vi "mainGUI_looped.vi"() -> ()   [LabVIEW 2025]
uses:
  <vilib>/Utility/error.llb/DialogType.ctl
  <vilib>/DAQmx/write.llb/DAQmx Write (Analog 1D Wfm NChan NSamp).vi
  <vilib>/DAQmx/read.llb/DAQmx Read (Analog Wfm 1Chan NSamp).vi
  <vilib>/DAQmx/read.llb/DAQmx Read (Counter U32 1Chan 1Samp).vi
  <vilib>/DAQmx/miscellaneous.llb/DAQmx Fill In Error Info.vi
  <vilib>/DAQmx/create/channels.llb/DAQmx Create Channel (CI-Count Edges).vi
  <vilib>/DAQmx/configure/trigger.llb/DAQmx Start Trigger (Digital Edge).vi
  <resource>/objmgr/daqmx.rc
  <vilib>/Analysis/NI_AALPro.lvlib
panel:
  in  "Run Live":bool caption="Run live"
  in  "Begin Experiment":bool
  in  "Connect Kinetix":bool
  in  "Run time":i32 caption="s" min=0
  in  "SLM default":bool
  in  "Load SLM image":bool
  in  "Create SLM image":bool
  in  "Save directory":path=path "D:/KinetixTest/SS_test"
  in  "# Trials":u32=1 caption="trials" min=1 step=1
  in  "Trial Time":dbl=0.1 caption="s" min=0.1 max=60.0 format="%#_2g"
  in  "Galvo frequency":u16(ring)=100 caption="Hz" items=["20"=20, "100"=100, "800"=800]
  in  "Galvo voltage":dbl=1.0 caption="V" min=0.1 max=1.8 format="%#_2g"
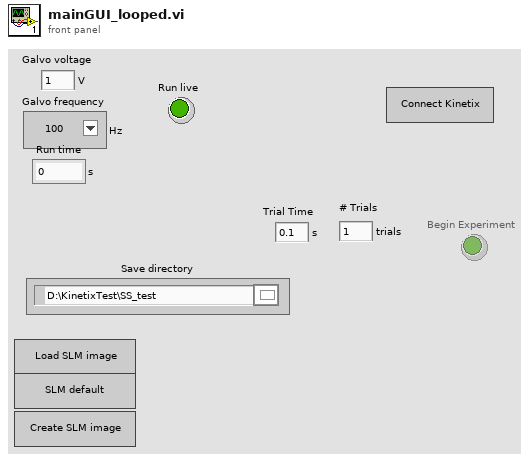
[diagram p1: front panel]
types:
  T1 = enum16{"open", "open or create", "create or replace", "create", "open (read-only)"}
  T2 = typedef "DialogType.ctl" = u16
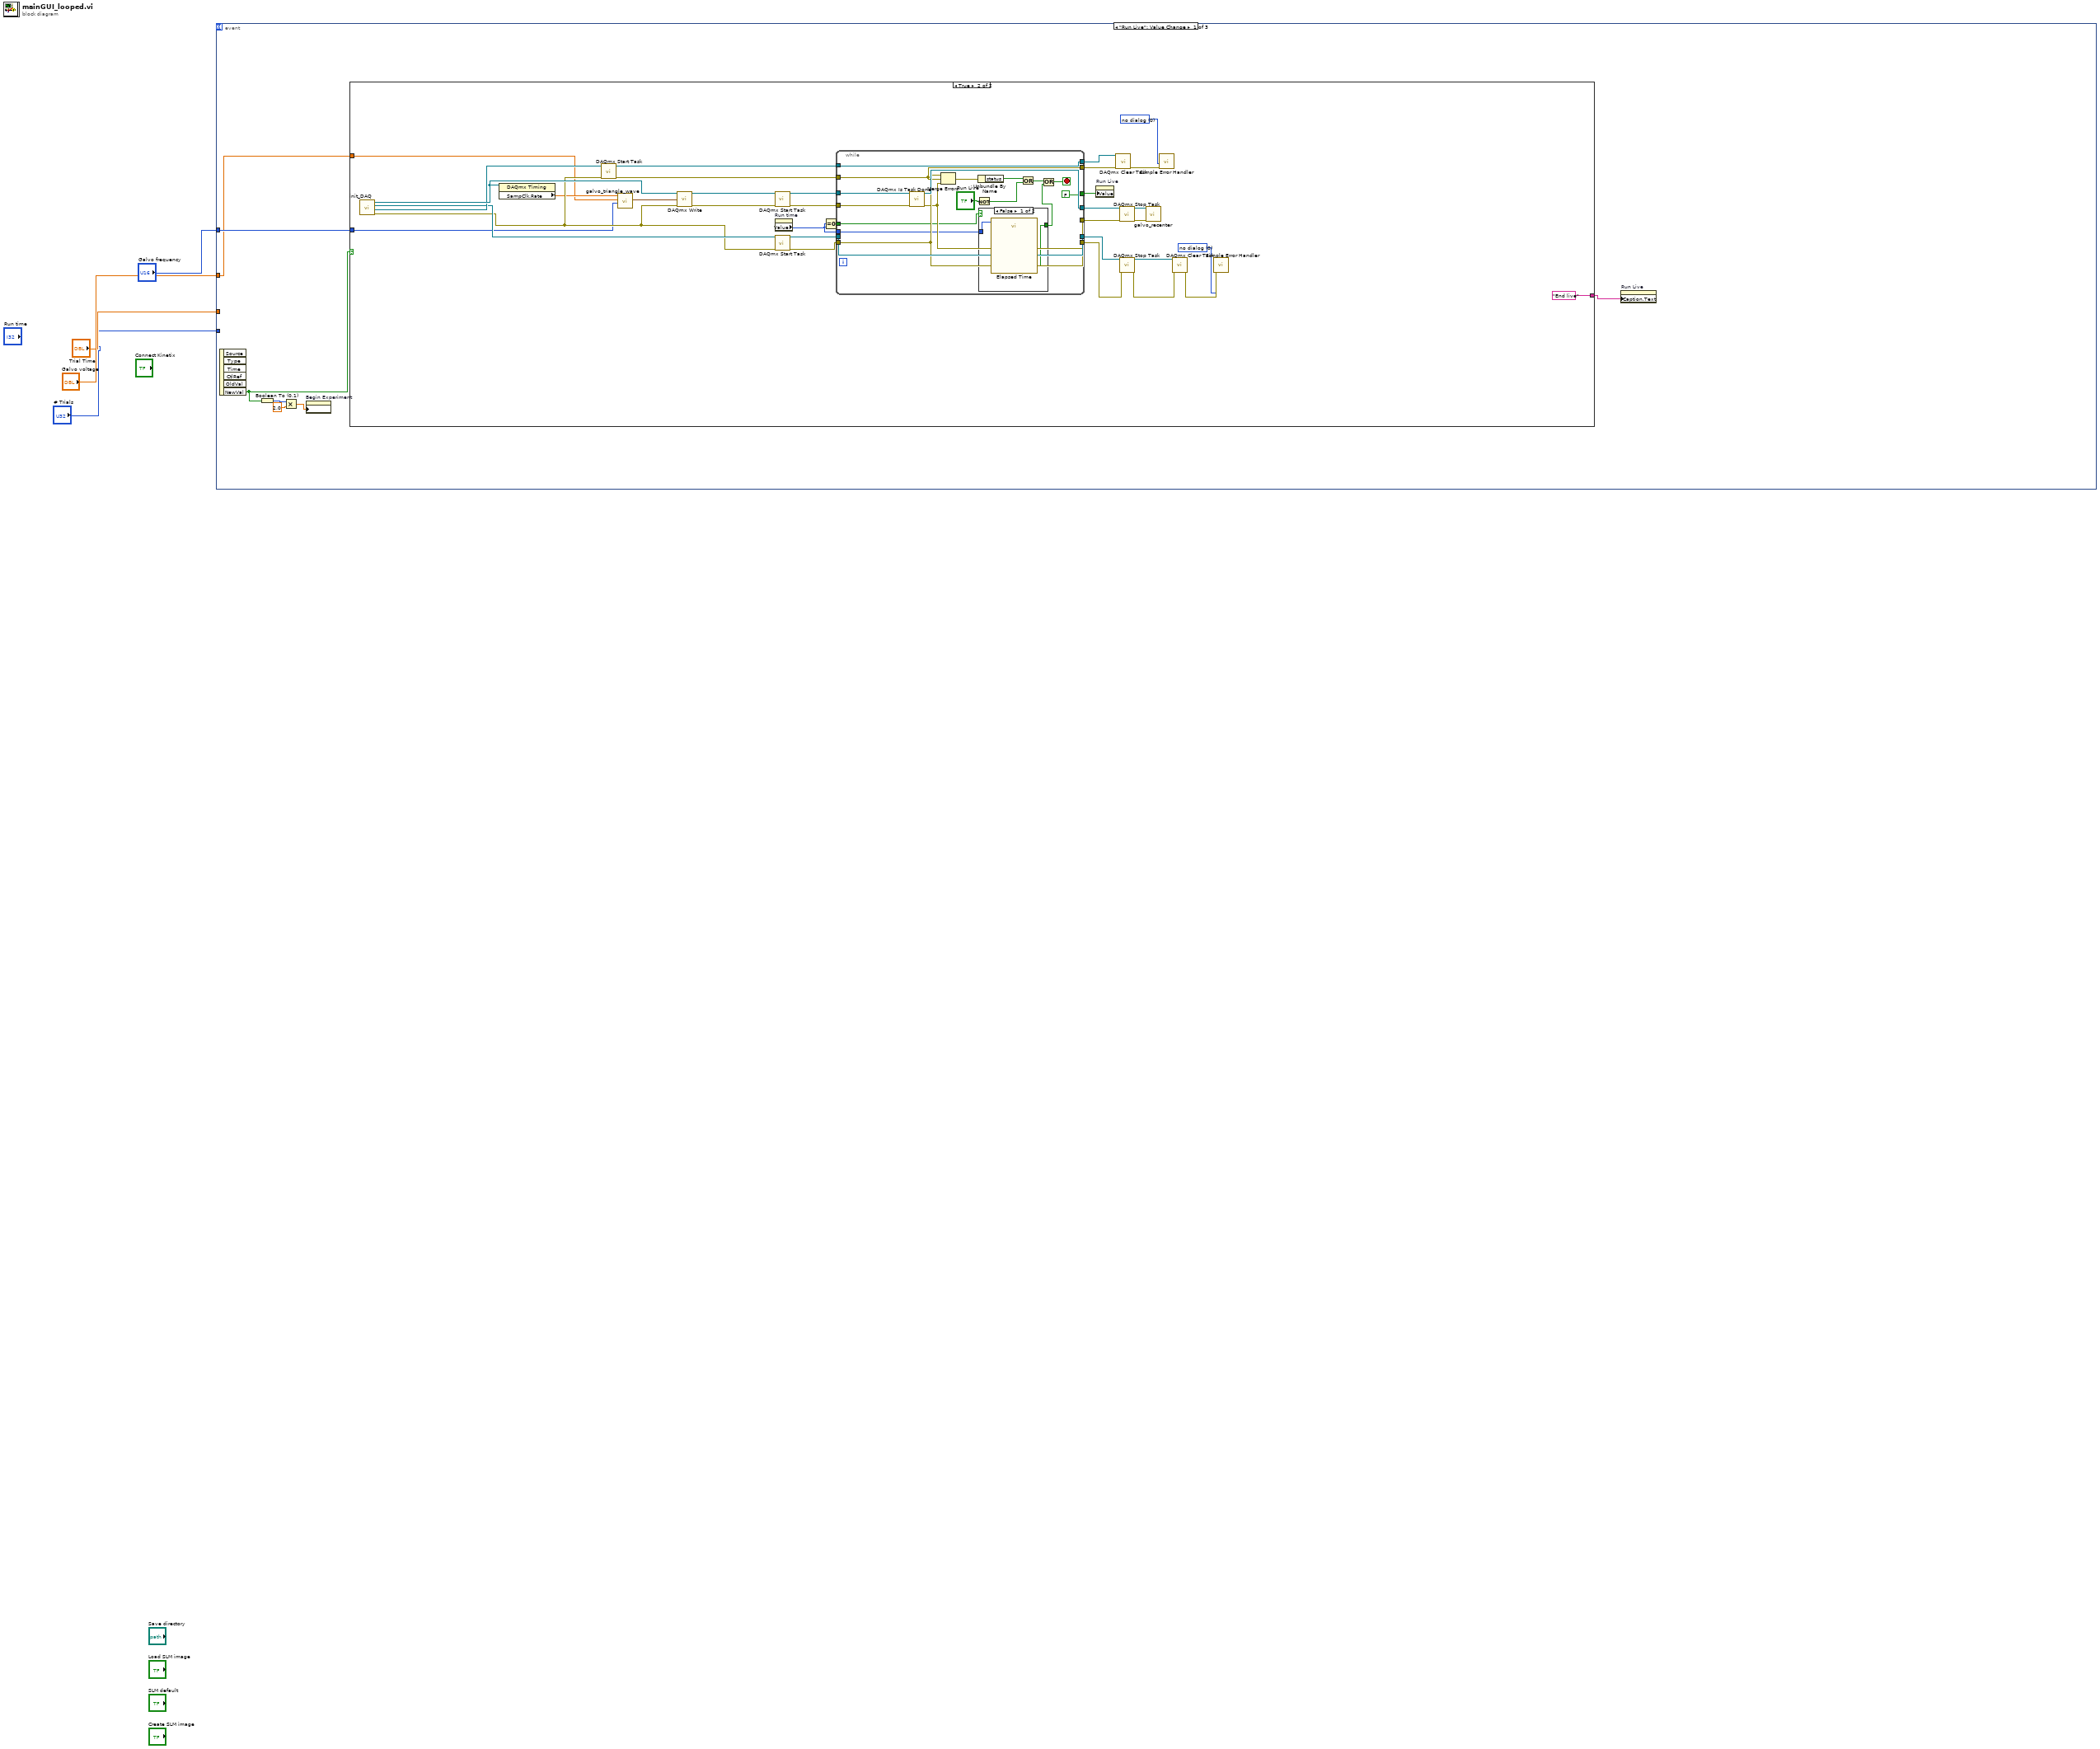
[diagram p0: block diagram]
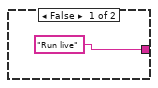
[diagram p2: hidden frame]
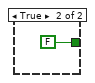
[diagram p3: hidden frame]
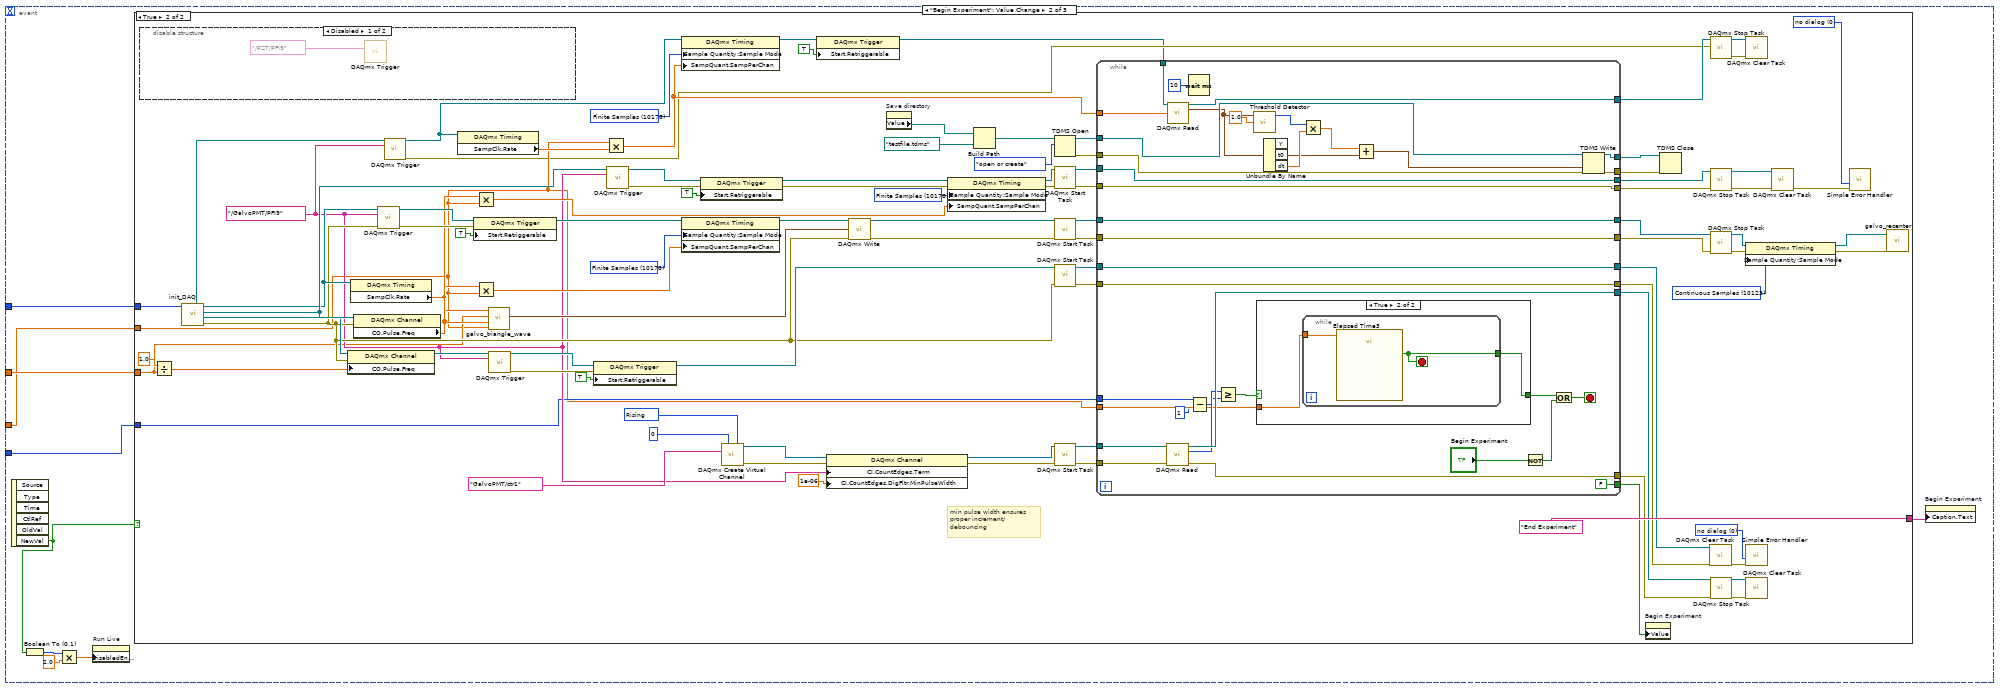
[diagram p4: hidden frame]
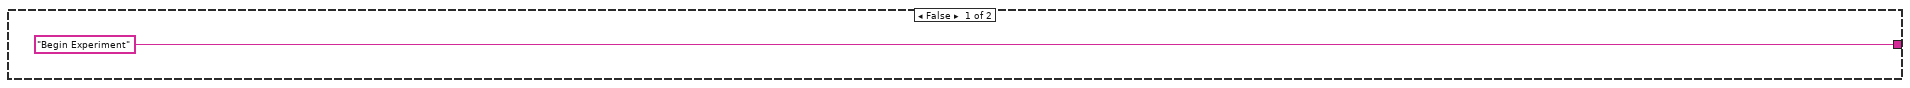
[diagram p5: hidden frame]
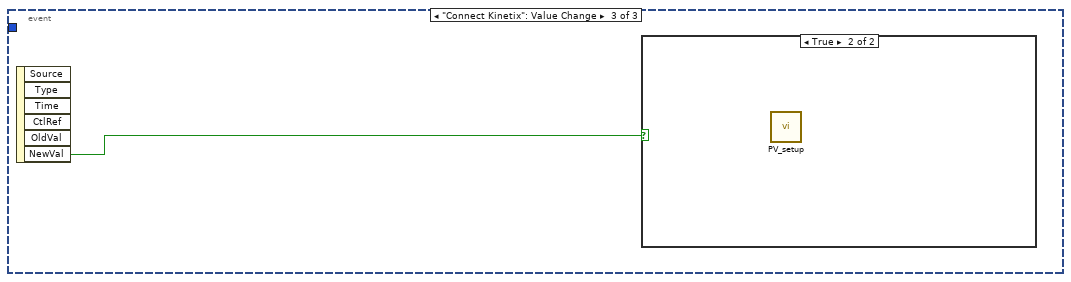
[diagram p8: hidden frame]
diagram:
  n1 = event shown="[0] \"Run Live\": Value Change" {
    selector: _ -> [_ _ _]
    dyn-events: _ -> [_ _ _]
    timeout: _ -> [_ _ _]
    tunnel: "Galvo frequency" -> [w7 w73 _]
    tunnel: "Galvo voltage" -> [w6 w72 _]
    tunnel: "Trial Time" -> [_ w71 _]
    tunnel: "# Trials" -> [_ w70 _]
    event "Run Live": Value Change {
      n2 = event-data() -> ("NewVal"=w5:bool)  [unwired: 1 in, 5 out]
      n3 = Boolean To (0,1)(Boolean=w5) -> (0, 1=w10:i16)
      n4 = Multiply(x=w10, y=2.0) -> (x*y=w9:dbl)
      n5 = property on="Begin Experiment" class="Bool (strict)"("DisabledEnum"=w9) -> ()  [unwired: 2 in, 2 out]
      n6 = case shown="True" w5 {
        tunnel: ["Run live" "End live"] -> w8
        tunnel: w7 -> [_ w14]
        tunnel: w6 -> [_ w13]
        frame False {
        }
        frame True {
          w33 = T2 0 items=["no dialog", "OK message", "continue or stop message", "OK message + warnings", "continue/stop + warnings"] ("type of dialog (OK msg:1)")
          w35 = T2 0 items=["no dialog", "OK message", "continue or stop message", "OK message + warnings", "continue/stop + warnings"] ("type of dialog (OK msg:1)")
          n7 = call "init_DAQ.vi"() -> ("error out"=w22:errorcluster, "shutter trigger task"=w28:refnum<k21>, "Kinetix trigger task"=w23:refnum<k21>, "galvo driving task"=w39:refnum<k21>)  [unwired: 7 in, 1 out]
          n8 = property class="DAQmx Timing"(reference=w39) -> ("SampClk.Rate"=w20:dbl)  [unwired: 1 in, 2 out]
          n9 = call <vilib>:"DAQmx Start Task.vi"("task/channels in"=w28, "error in"=w22) -> ("task out"=w32:refnum<k21>, "error out"=w30:errorcluster)  [unwired: 12 in]
          n10 = call "galvo_triangle_wave.vi"("final frequency"=w14, "amplitude"=w13, "sample rate"=w20) -> ("waveform array out"=w21:waveform(dbl)[])  [unwired: 8 in]
          n11 = call-poly <vilib>:"DAQmx Write.vi"("task/channels in"=w39, "data"=w21, "error in"=w22) -> ("task out"=w45:refnum<k21>, "error out"=w44:errorcluster)  [unwired: 10 in, 1 out]
          n12 = call <vilib>:"DAQmx Start Task.vi"("task/channels in"=w45, "error in"=w44) -> ("task out"=w40:refnum<k21>, "error out"=w41:errorcluster)  [unwired: 12 in]
          n13 = property on="Run time" class="DigNum (strict)"() -> ("Value"=w16:i32)  [unwired: 2 in, 2 out]
          n14 = call <vilib>:"DAQmx Start Task.vi"("task/channels in"=w23, "error in"=w22) -> ("task out"=w38:refnum<k21>, "error out"=w37:errorcluster)  [unwired: 12 in]
          n15 = Equal To 0?(x=w16) -> (x = 0?=w17:bool)
          n16 = while {
            tunnel: w40 -> [w64]
            tunnel: w41 -> [w63]
            tunnel: [w53] -> w43
            tunnel: [w62] -> w42
            tunnel: w38 -> [w60]
            tunnel: w37 -> [w55]
            tunnel: [w55] -> w27
            tunnel: [w60] -> w25
            tunnel: w32 -> [w57]
            tunnel: [w57] -> w31
            tunnel: w30 -> [w54]
            tunnel: [w54] -> w29
            tunnel: w17 -> [w50]
            tunnel: w16 -> [w49]
            tunnel: [FALSE] -> w15
            stop <- w48 stop-if-true
            n17 = call <vilib>:"DAQmx Is Task Done.vi"("task/channels in"=w64, "error in"=w63) -> ("task out"=w62:refnum<k21>, "error out"=w53:errorcluster)  [unwired: 11 in, 1 out]
            n18 = Merge Errors(w55, w54, w53) -> (w56:errorcluster)
            n19 = Not(x="Run Live") -> (.not. x?=w59:bool)
            n20 = Unbundle By Name(w56) -> ("status"=w61:bool)
            n21 = case shown="False" w50 {
              tunnel: [w66 FALSE] -> w51
              tunnel: w49 -> [w65 _]
              frame False {
                n22 = call "Elapsed Time"("Time Target (s)"=w65) -> ("Time has Elapsed"=w66:bool)  [unwired: 11 in, 7 out]
              }
              frame True {
              }
            }
            n23 = Or(x=w61, y=w59) -> (x .or. y?=w52:bool)
            n24 = Or(x=w52, y=w51) -> (x .or. y?=w48:bool)
          }
          n25 = property on="Run Live" class="Bool (strict)"("Value"=w15) -> ()  [unwired: 2 in, 2 out]
          n26 = call <vilib>:"DAQmx Clear Task.vi"("task in"=w31, "error in"=w29) -> ("error out"=w34:errorcluster)  [unwired: 13 in]
          n27 = call <vilib>:"DAQmx Stop Task.vi"("task/channels in"=w42, "error in"=w43) -> ("task out"=w19:refnum<k21>, "error out"=w18:errorcluster)  [unwired: 12 in]
          n28 = call <vilib>:"DAQmx Stop Task.vi"("task/channels in"=w25, "error in"=w27) -> ("task out"=w24:refnum<k21>, "error out"=w26:errorcluster)  [unwired: 12 in]
          n29 = call "galvo_recenter.vi"("error in"=w18, "task/channels in"=w19) -> ()  [unwired: 10 in]
          n30 = call <vilib>:"Simple Error Handler.vi"("type of dialog (OK msg:1)"=w33, "error in (no error)"=w34) -> ()  [unwired: 3 in, 5 out]
          n31 = call <vilib>:"DAQmx Clear Task.vi"("task in"=w24, "error in"=w26) -> ("error out"=w36:errorcluster)  [unwired: 13 in]
          n32 = call <vilib>:"Simple Error Handler.vi"("type of dialog (OK msg:1)"=w35, "error in (no error)"=w36) -> ()  [unwired: 3 in, 5 out]
        }
      }
      n33 = property on="Run Live" class="Bool (strict)"("Caption.Text"=w8) -> ()  [unwired: 2 in, 2 out]
    }
    event "Begin Experiment": Value Change {
      n34 = event-data() -> ("NewVal"=w74:bool)  [unwired: 1 in, 5 out]
      n35 = Boolean To (0,1)(Boolean=w74) -> (0, 1=w75:i16)
      n36 = Multiply(x=w75, y=2.0) -> (x*y=w68:dbl)
      n37 = property on="Run Live" class="Bool (strict)"("DisabledEnum"=w68) -> ()  [unwired: 2 in, 2 out]
      n38 = case shown="True" w74 {
        tunnel: ["Begin Experiment" "End Experiment"] -> w69
        tunnel: w73 -> [_ w83]
        tunnel: w72 -> [_ w81]
        tunnel: w70 -> [_ w82]
        tunnel: w71 -> [_ w80]
        frame False {
        }
        frame True {
          w86 = 10178 items=["Finite Samples"=10178, "Continuous Samples"=10123, "Hardware Timed Single Point"=12522] ("SampQuant.SampMode")
          w99 = 10178 items=["Finite Samples"=10178, "Continuous Samples"=10123, "Hardware Timed Single Point"=12522] ("SampQuant.SampMode")
          w106 = 10123 items=["Finite Samples"=10178, "Continuous Samples"=10123, "Hardware Timed Single Point"=12522] ("SampQuant.SampMode")
          w133 = 10280 items=["Rising"=10280, "Falling"=10171] ("edge")
          w105 = tag "/GalvoPMT/PFI9" ("source")
          w113 = 10178 items=["Finite Samples"=10178, "Continuous Samples"=10123, "Hardware Timed Single Point"=12522] ("SampQuant.SampMode")
          w169 = T2 0 items=["no dialog", "OK message", "continue or stop message", "OK message + warnings", "continue/stop + warnings"] ("type of dialog (OK msg:1)")
          w171 = T2 0 items=["no dialog", "OK message", "continue or stop message", "OK message + warnings", "continue/stop + warnings"] ("type of dialog (OK msg:1)")
          # "min pulse width ensures proper increment/debouncing"
          n39 = disable-structure shown="Disabled" {
            frame Disabled {
              n40 = call-poly <vilib>:"DAQmx Trigger.vi"("source"=tag "/PZT/PFI9") -> ()  [unwired: 13 in, 2 out]
            }
            frame Enabled {
            }
          }
          n41 = Divide(x=1.0, y=w81) -> (x/y=w129:dbl)
          n42 = call "init_DAQ.vi"("Frame frequency"=w83) -> ("error out"=w118:errorcluster, "shutter trigger task"=w131:refnum<k21>, "Kinetix trigger task"=w150:refnum<k21>, "galvo driving task"=w119:refnum<k21>, "Kinetix timing read task"=w104:refnum<k21>)  [unwired: 6 in]
          n43 = property class="DAQmx Channel"(reference=w131, error in=w118, "CO.Pulse.Freq"=w129) -> (reference out=w132:refnum<k21>)  [unwired: 1 out]
          n44 = property class="DAQmx Timing"(reference=w119) -> ("SampClk.Rate"=w109:dbl)  [unwired: 1 in, 2 out]
          n45 = property class="DAQmx Channel"(reference=w150, error in=w118) -> ("CO.Pulse.Freq"=w111:dbl)  [unwired: 2 out]
          n46 = call-poly <vilib>:"DAQmx Trigger.vi"("task/channels in"=w119, "source"=w105, "error in"=w118) -> ("task out"=w166:refnum<k21>, "error out"=w165:errorcluster)  [unwired: 11 in]
          n47 = call-poly <vilib>:"DAQmx Trigger.vi"("task/channels in"=w104, "source"=w105) -> ("task out"=w90:refnum<k21>, "error out"=w79:errorcluster)  [unwired: 12 in]
          n48 = property class="DAQmx Timing"(reference=w90) -> ("SampClk.Rate"=w91:dbl)  [unwired: 1 in, 2 out]
          n49 = property class="DAQmx Trigger"(reference=w166, error in=w165, "Start.Retriggerable"=TRUE) -> (reference out=w120:refnum<k21>)  [unwired: 1 out]
          n50 = Multiply(x=w111, y=w80) -> (x*y=w110:dbl)
          n51 = Multiply(x=w109, y=w80) -> (x*y=w112:dbl)
          n52 = call "galvo_triangle_wave.vi"("trial seconds"=w80, "final frequency"=w111, "amplitude"=w81, "sample rate"=w109) -> ("waveform array out"=w126:waveform(dbl)[])  [unwired: 7 in]
          n53 = call-poly <vilib>:"DAQmx Trigger.vi"("task/channels in"=w132, "source"=w105) -> ("task out"=w148:refnum<k21>, "error out"=w149:errorcluster)  [unwired: 12 in]
          n54 = property class="DAQmx Trigger"(reference=w148, error in=w149, "Start.Retriggerable"=TRUE) -> (reference out=w147:refnum<k21>)  [unwired: 1 out]
          n55 = Multiply(x=w80, y=w91) -> (x*y=w89:dbl)
          n56 = call-poly <vilib>:"DAQmx Trigger.vi"("task/channels in"=w150, "source"=w105) -> ("task out"=w152:refnum<k21>, "error out"=w151:errorcluster)  [unwired: 12 in]
          n57 = property class="DAQmx Timing"(reference=w90, "Sample Quantity:Sample Mode"=w99, "SampQuant.SampPerChan"=w89) -> (reference out=w88:refnum<k21>)  [unwired: 1 in, 1 out]
          n58 = property class="DAQmx Timing"(reference=w120, "Sample Quantity:Sample Mode"=w113, "SampQuant.SampPerChan"=w112) -> (reference out=w121:refnum<k21>)  [unwired: 1 in, 1 out]
          n59 = property class="DAQmx Trigger"(reference=w152, error in=w151, "Start.Retriggerable"=TRUE) -> (reference out=w114:refnum<k21>, error out=w115:errorcluster)
          n60 = call-poly <vilib>:"DAQmx Create Virtual Channel.vi"("initial count"=u32 0, "edge"=w133, "counter"=tag "GalvoPMT/ctr1") -> ("task out"=w163:refnum<k21>, "error out"=w162:errorcluster)  [unwired: 11 in]
          n61 = property class="DAQmx Trigger"(reference=w88, "Start.Retriggerable"=TRUE) -> (reference out=w78:refnum<k21>)  [unwired: 1 in, 1 out]
          n62 = property class="DAQmx Channel"(reference=w163, error in=w162, "CI.CountEdges.Term"=w105, "CI.CountEdges.DigFltr.MinPulseWidth"=1e-06 ("DI.DigFltr.MinPulseWidth")) -> (reference out=w156:refnum<k21>, error out=w155:errorcluster)
          n63 = call-poly <vilib>:"DAQmx Write.vi"("task/channels in"=w121, "data"=w126, "error in"=w118) -> ("task out"=w125:refnum<k21>, "error out"=w124:errorcluster)  [unwired: 10 in, 1 out]
          n64 = property on="Save directory" class="Path"() -> ("Value"=w103:path)  [unwired: 2 in, 2 out]
          n65 = property class="DAQmx Timing"(reference=w114, error in=w115, "Sample Quantity:Sample Mode"=w86, "SampQuant.SampPerChan"=w110) -> (reference out=w117:refnum<k21>, error out=w116:errorcluster)
          n66 = Build Path(base path=w103, name or relative path=path "testfile.tdms") -> (appended path=w98:path)
          n67 = TDMS Open(10:T1."open or create" ("operation (0:open)"), 11:w98) -> (0:w95:errorcluster, 3:w97:refnum<k34>)  [unwired: 5 in]
          n68 = call <vilib>:"DAQmx Start Task.vi"("task/channels in"=w117, "error in"=w116) -> ("task out"=w142:refnum<k21>, "error out"=w141:errorcluster)  [unwired: 12 in]
          n69 = call <vilib>:"DAQmx Start Task.vi"("task/channels in"=w125, "error in"=w124) -> ("task out"=w123:refnum<k21>, "error out"=w122:errorcluster)  [unwired: 12 in]
          n70 = call <vilib>:"DAQmx Start Task.vi"("task/channels in"=w147, "error in"=w118) -> ("task out"=w138:refnum<k21>, "error out"=w135:errorcluster)  [unwired: 12 in]
          n71 = call <vilib>:"DAQmx Start Task.vi"("task/channels in"=w156, "error in"=w155) -> ("task out"=w154:refnum<k21>, "error out"=w153:errorcluster)  [unwired: 12 in]
          n72 = while {
            tunnel: w82 -> [w177]
            tunnel: [w208] -> w160
            tunnel: [w207] -> w158
            tunnel: w154 -> [w204]
            tunnel: w153 -> [w203]
            tunnel: [w197] -> w144
            tunnel: [w194] -> w143
            tunnel: w142 -> [w201]
            tunnel: w141 -> [w202]
            tunnel: [w202] -> w140
            tunnel: [w201] -> w139
            tunnel: w138 -> [w193]
            tunnel: [w193] -> w137
            tunnel: [w200] -> w136
            tunnel: w135 -> [w200]
            tunnel: [FALSE] -> w128
            tunnel: w123 -> [w194]
            tunnel: w122 -> [w197]
            tunnel: w80 -> [w192]
            tunnel: w97 -> [w190]
            tunnel: [w189] -> w96
            tunnel: w95 -> [w191]
            tunnel: [w188] -> w94
            tunnel: [w187] -> w93
            tunnel: w89 -> [w186]
            tunnel: w78 -> [w175]
            stop <- w199 stop-if-true
            n73 = call-poly <vilib>:"DAQmx Read.vi"("task/channels in"=w204, "error in"=w203) -> ("task out"=w208:refnum<k21>, "data"=w206:u32, "error out"=w207:errorcluster)  [unwired: 11 in]
            n74 = call-poly <vilib>:"DAQmx Read.vi"("task/channels in"=w175, "number of samples per channel"=w186) -> ("task out"=w187:refnum<k21>, "data"=w179:waveform(dbl))  [unwired: 11 in, 1 out]
            n75 = Wait (ms)(milliseconds to wait=u32 10) -> ()  [unwired: 1 out]
            n76 = Subtract(x=w177, y=u32 1) -> (x-y=w176:u32)
            n77 = Greater Or Equal?(x=w206, y=w176) -> (x >= y?=w196:bool)
            n78 = call <vilib>:"Threshold Detector.vi"("threshold"=1.0, "X"=w179) -> ("Indices"=w184:i32[])  [unwired: 1 in, 2 out]
            n79 = case shown="True" w196 {
              selector: w196 -> [w211 _]
              tunnel: [w211 w213] -> w195
              tunnel: w192 -> [_ w212]
              frame False {
              }
              frame True {
                n80 = while {
                  tunnel: [w214] -> w213
                  tunnel: w212 -> [w215]
                  stop <- w214 stop-if-true
                  n81 = call "Elapsed Time3"("Time Target (s)"=w215) -> ("Time has Elapsed"=w214:bool)  [unwired: 11 in, 7 out]
                }
              }
            }
            n82 = Unbundle By Name(w179) -> ("t0"=w180:timestamp, "dt"=w183:dbl)  [unwired: 1 out]
            n83 = Multiply(x=w184, y=w183) -> (x*y=w182:dbl[])
            n84 = Add(x=w182, y=w180) -> (x+y=w185:timestamp[])
            n85 = Not(x="Begin Experiment") -> (.not. x?=w209:bool)
            n86 = Or(x=w195, y=w209) -> (x .or. y?=w199:bool)
            n87 = TDMS Write(0:w190, 9:w185, 11:w191) -> (4:w189:refnum<k34>, 15:w188:errorcluster)  [unwired: 3 in, 2 out]
          }
          n88 = property on="Begin Experiment" class="Bool (strict)"("Value"=w128) -> ()  [unwired: 2 in, 2 out]
          n89 = TDMS Close(8:w94, 11:w96) -> ()  [unwired: 2 out]
          n90 = call <vilib>:"DAQmx Clear Task.vi"("task in"=w137, "error in"=w136) -> ("error out"=w170:errorcluster)  [unwired: 13 in]
          n91 = call <vilib>:"DAQmx Stop Task.vi"("task/channels in"=w93, "error in"=w79) -> ("task out"=w101:refnum<k21>, "error out"=w100:errorcluster)  [unwired: 12 in]
          n92 = call <vilib>:"DAQmx Stop Task.vi"("task/channels in"=w139, "error in"=w140) -> ("task out"=w167:refnum<k21>, "error out"=w168:errorcluster)  [unwired: 12 in]
          n93 = call <vilib>:"DAQmx Stop Task.vi"("task/channels in"=w143, "error in"=w144) -> ("task out"=w108:refnum<k21>, "error out"=w107:errorcluster)  [unwired: 12 in]
          n94 = call <vilib>:"DAQmx Stop Task.vi"("task/channels in"=w160, "error in"=w158) -> ("task out"=w159:refnum<k21>, "error out"=w157:errorcluster)  [unwired: 12 in]
          n95 = call <vilib>:"DAQmx Clear Task.vi"("task in"=w101, "error in"=w100) -> ()  [unwired: 13 in, 1 out]
          n96 = property class="DAQmx Timing"(reference=w108, error in=w107, "Sample Quantity:Sample Mode"=w106) -> (reference out=w85:refnum<k21>, error out=w84:errorcluster)
          n97 = call <vilib>:"Simple Error Handler.vi"("type of dialog (OK msg:1)"=w169, "error in (no error)"=w170) -> ()  [unwired: 3 in, 5 out]
          n98 = call <vilib>:"DAQmx Clear Task.vi"("task in"=w159, "error in"=w157) -> ()  [unwired: 13 in, 1 out]
          n99 = call <vilib>:"DAQmx Clear Task.vi"("task in"=w167, "error in"=w168) -> ("error out"=w172:errorcluster)  [unwired: 13 in]
          n100 = call <vilib>:"Simple Error Handler.vi"("type of dialog (OK msg:1)"=w171, "error in (no error)"=w172) -> ()  [unwired: 3 in, 5 out]
          n101 = call "galvo_recenter.vi"("error in"=w84, "task/channels in"=w85) -> ()  [unwired: 10 in]
        }
      }
      n102 = property on="Begin Experiment" class="Bool (strict)"("Caption.Text"=w69) -> ()  [unwired: 2 in, 2 out]
    }
    event "Connect Kinetix": Value Change {
      n103 = event-data() -> ("NewVal"=w216:bool)  [unwired: 1 in, 5 out]
      n104 = case shown="True" w216 {
        frame False {
        }
        frame True {
          n105 = call "PV_setup.vi"() -> ()  [unwired: 9 in, 3 out]
        }
      }
    }
  }
